vi "Stimulus.Run.vi"(8 "error in (no error)":errorcluster, 11 "Cluster in":T1) -> (0 "error out":errorcluster, 3 "Cluster out":T1)   [LabVIEW 2013, in "Simple Sequence Tools - Execution.lvlib"]
uses:
  Simple Sequence Tools - Execution.lvlib
  Types/Main.StateVariables.ctl
  Types/Execute.UserEventRefs.ctl
  <vilib>/NI Veristand/Execution/Workspace/SystemStateRegEventRef.ctl
  Types/Execution.SequenceState.ctl
  <vilib>/NI Veristand/Execution/DataLogging/DataLoggingSpecification Ref.ctl
  NationalInstruments.VeriStand.ClientAPI
  <vilib>/NI Veristand/Execution/DataLogging/IDataLogging Ref.ctl
  <vilib>/NI Veristand/Execution/Workspace/WorkspaceAPI.ctl
  NationalInstruments.VeriStand.RealTimeSequenceDefinitionApi
  <vilib>/NI Veristand/Execution/Workspace/SystemStateEventRef.ctl
  Shared/Types/INI.Settings
  <vilib>/NI Veristand/Execution/DataLogging/NI_VS Data Logging API.lvlib
  <vilib>/NI Veristand/Execution/Workspace/NI_VS Workspace ExecutionAPI.lvlib
  Shared/Simple Sequence Tools - Shared.lvlib
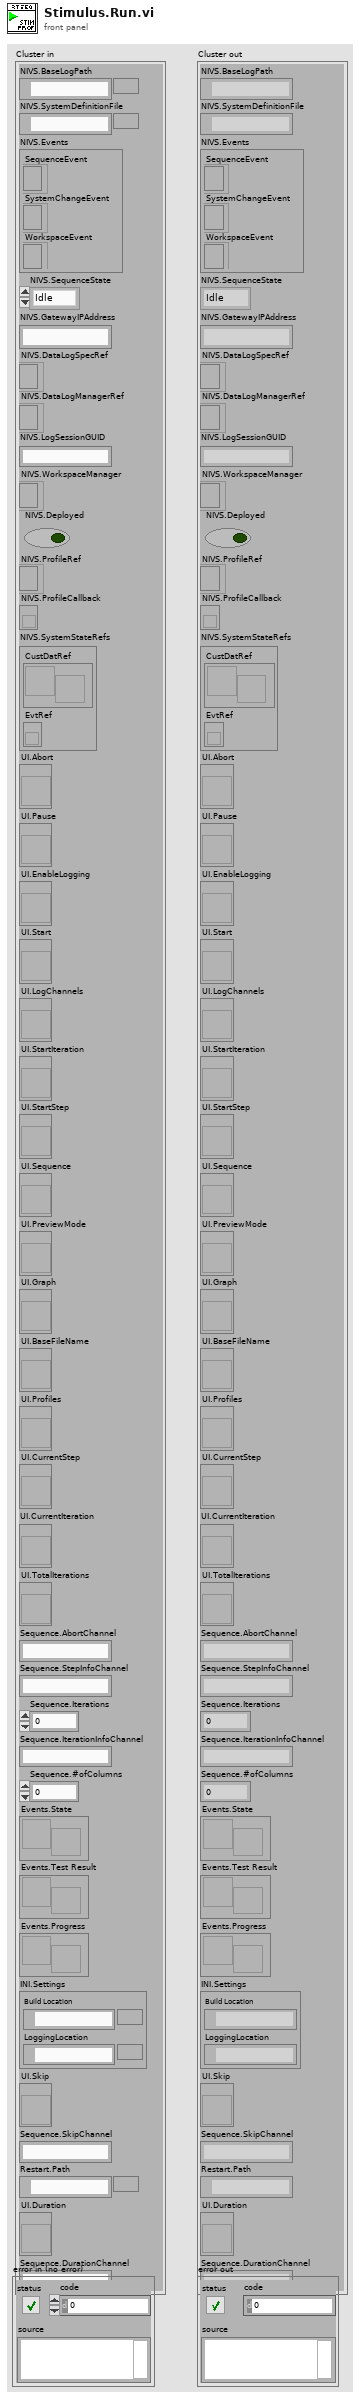
[diagram p1: front panel]
types:
  T1 = typedef "Simple Sequence Tools - Execution.lvlib/Main.StateVariables.ctl" = cluster{"NIVS.BaseLogPath":path, "NIVS.SystemDefinitionFile":path, "NIVS.Events":T2, "NIVS.SequenceState":T4, "NIVS.GatewayIPAddress":string, "NIVS.DataLogSpecRef":T5, "NIVS.DataLogManagerRef":T6, "NIVS.LogSessionGUID":string, "NIVS.WorkspaceManager":T7, "NIVS.Deployed":bool, "NIVS.ProfileRef":refnum<k24>, "NIVS.ProfileCallback":refnum<k27>, "NIVS.SystemStateRefs":T8, "UI.Abort":refnum<vi>, "UI.Pause":refnum<vi>, "UI.EnableLogging":refnum<vi>, "UI.Start":refnum<vi>, "UI.LogChannels":refnum<vi>, "UI.StartIteration":refnum<vi>, "UI.StartStep":refnum<vi>, "UI.Sequence":refnum<vi>, "UI.PreviewMode":refnum<vi>, "UI.Graph":refnum<vi>, "UI.BaseFileName":refnum<vi>, "UI.Profiles":refnum<vi>, "UI.CurrentStep":refnum<vi>, "UI.CurrentIteration":refnum<vi>, "UI.TotalIterations":refnum<vi>, "Sequence.AbortChannel":string, "Sequence.StepInfoChannel":string, "Sequence.Iterations":u32, "Sequence.IterationInfoChannel":string, "Sequence.#ofColumns":i32, "Events.State":refnum<user-event>, "Events.Test Result":refnum<user-event>, "Events.Progress":refnum<user-event>, "INI.Settings":T9, "UI.Skip":refnum<vi>, "Sequence.SkipChannel":string, "Restart.Path":path, "UI.Duration":refnum<vi>, "Sequence.DurationChannel":string}
  T2 = typedef "Simple Sequence Tools - Execution.lvlib/Execute.UserEventRefs.ctl" = cluster{"SequenceEvent":refnum<event-registration>, "SystemChangeEvent":T3, "WorkspaceEvent":refnum<event-registration>}
  T3 = typedef "NI_VS Workspace ExecutionAPI.lvlib/SystemStateRegEventRef.ctl" = refnum<event-registration>
  T4 = typedef "Simple Sequence Tools - Execution.lvlib/Execution.SequenceState.ctl" = enum16{"Idle", "Initializing", "Running", "Paused", "Finalizing", "Complete"}
  T5 = typedef "NI_VS Data Logging API.lvlib/DataLoggingSpecification Ref.ctl" = refnum<k24>
  T6 = typedef "NI_VS Data Logging API.lvlib/IDataLogging Ref.ctl" = refnum<k24>
  T7 = typedef "NI_VS Workspace ExecutionAPI.lvlib/WorkspaceAPI.ctl" = refnum<k24>
  T8 = typedef "NI_VS Workspace ExecutionAPI.lvlib/SystemStateEventRef.ctl" = cluster{"CustDatRef":refnum<user-event>, "EvtRef":refnum<k27>}
  T9 = typedef "Simple Sequence Tools - Shared.lvlib/INI.Settings" = cluster{"Build Location":path, "LoggingLocation":path}
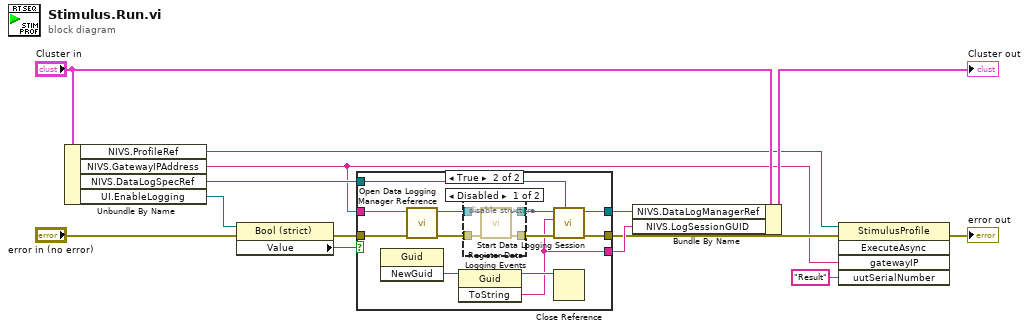
[diagram p0: block diagram]
diagram:
  n1 = Unbundle By Name("Cluster in") -> ("NIVS.ProfileRef"=w1:refnum<k24>, "NIVS.GatewayIPAddress"=w4:string, "NIVS.DataLogSpecRef"=w13:T5, "UI.EnableLogging"=w8:refnum<vi>)
  n2 = property class="Bool (strict)"(reference=w8, error in="error in (no error)") -> (error out=w7:errorcluster, "Value"=w9:bool)  [unwired: 1 out]
  n3 = case shown="True" w9 {
    tunnel: w7 -> [w15 w27]
    tunnel: w4 -> [_ w26]
    tunnel: w13 -> [_ w25]
    tunnel: [w15 w20] -> w5
    tunnel: [_ w19] -> w10
    tunnel: [_ w16] -> w14
    frame False {
    }
    frame True {
      n4 = invoke class="Guid" method="NewGuid"() -> ("NewGuid"=w18:refnum<k24>)  [unwired: 3 in, 2 out]
      n5 = call <vilib>:"Open Data Logging Manager Reference.vi"("error in (no error)"=w27, "Gateway IP Address (\"\": localhost)"=w26) -> ("error out"=w24:errorcluster, "Data Logging Manager Ref out"=w23:T6)  [unwired: 8 in]
      n6 = invoke class="Guid" method="ToString"(reference=w18) -> (reference out=w17:refnum<k24>, "ToString"=w16:string)  [unwired: 2 in, 1 out]
      n7 = disable-structure shown="Disabled" {
        disable-tunnel: w24 -> [w31 w33]
        disable-tunnel: w23 -> [w30 w32]
        disable-tunnel: [w29 w33] -> w22
        disable-tunnel: [w28 w32] -> w21
        frame Disabled {
          n8 = call <vilib>:"Register Data Logging Events.vi"("error in (no error)"=w31, "Data Logging Manager Ref in"=w30) -> ("error out"=w29:errorcluster, "Data Logging Manager Ref out"=w28:T6)  [unwired: 6 in, 2 out]
        }
        frame Enabled {
        }
      }
      n9 = call <vilib>:"Start Data Logging Session.vi"("Data Logging Specification Ref in"=w25, "error in (no error)"=w22, "Session Name in"=w16, "Data Logging Manager Ref in"=w21) -> ("error out"=w20:errorcluster, "Data Logging Manager Ref out"=w19:T6)  [unwired: 5 in, 1 out]
      n10 = Close Reference(reference=w17) -> ()  [unwired: 1 in, 1 out]
    }
  }
  n11 = Bundle By Name(cluster="Cluster in", "NIVS.DataLogManagerRef"=w10, "NIVS.LogSessionGUID"=w14) -> (→"Cluster out":T1)
  n12 = invoke class="StimulusProfile" method="ExecuteAsync"(reference=w1, error in=w5, "gatewayIP"=w4, "uutSerialNumber"="Result") -> (error out=→"error out":errorcluster)  [unwired: 1 in, 4 out]
